vi "test.add.data.to.buffer.vi"() -> (3 "All Passed":bool)   [LabVIEW 2022 SP3]
uses:
  buffer.test.case.ctl
  data.ctl
  <vilib>/rvi/Emulation/niFpgaGetClockAttributes.vi
  <vilib>/rvi/Emulation/niFpgaSctlEmulationGetInTimedLoop.vi
  <vilib>/rvi/Emulation/niFpgaEmulationReportErrorSimple.vi
  <vilib>/rvi/Emulation/niFpgaCriticalErrorInLSC.vi
panel:
  in  "Test Case #12 - Buffer has 16 elements, Data has 3 elements":T1={"data.valid"=TRUE, "data"={"enabled"=[TRUE, TRUE, TRUE, FALSE, FALSE, FALSE, FALSE, FALSE], "byte"=[1, 2, 3, 4, 5, 6, 7, 0]}, "buffer"=[1234605616436508552, 48057234611961600, 0, 0, 0, 0, 0, 0, 0], "buffer.length"=16, "exp.buffer.value.1"=72623842526232576, "index 1"=2, "exp.buffer.value.2"=0, "index 2"=3, "exp.buffer.length"=19} {"exp.buffer.value.2" format="%.0x"; "index 1" format="%.0x"; "exp.buffer.value.1" format="%.0x"; "buffer" format="%.0x"; "data"."byte" format="%.0x"}
  out "Passed 12":bool
  in  "Test Case #11 - Buffer has 16 elements, Data has 8 elements":T1={"data.valid"=TRUE, "data"={"enabled"=[TRUE, TRUE, TRUE, TRUE, TRUE, TRUE, TRUE, TRUE], "byte"=[1, 2, 3, 4, 5, 6, 7, 8]}, "buffer"=[1234605616436508552, 48057234611961600, 0, 0, 0, 0, 0, 0, 0], "buffer.length"=16, "exp.buffer.value.1"=72623859790382856, "index 1"=2, "exp.buffer.value.2"=0, "index 2"=3, "exp.buffer.length"=24} {"exp.buffer.value.2" format="%.0x"; "index 1" format="%.0x"; "exp.buffer.value.1" format="%.0x"; "buffer" format="%.0x"; "data"."byte" format="%.0x"}
  out "Passed 11":bool
  in  "Test Case #10 - Buffer has 32 elements, Data has 8 elements":T1={"data.valid"=TRUE, "data"={"enabled"=[TRUE, TRUE, TRUE, TRUE, TRUE, TRUE, TRUE, TRUE], "byte"=[34, 255, 255, 255, 255, 255, 255, 255]}, "buffer"=[1234605616436508552, 48057234611961600, 1234605616436508552, 11024811887802974208, 0, 0, 0, 0, 0], "buffer.length"=32, "exp.buffer.value.1"=2522015791327477759, "index 1"=4, "exp.buffer.value.2"=0, "index 2"=5, "exp.buffer.length"=40} {"exp.buffer.value.2" format="%.0x"; "index 1" format="%.0x"; "exp.buffer.value.1" format="%.0x"; "buffer" format="%.0x"; "data"."byte" format="%.0x"}
  out "Passed 10":bool
  in  "Test Case #9 - Buffer has 26 elements, Data has 1 element":T1={"data.valid"=TRUE, "data"={"enabled"=[TRUE, FALSE, FALSE, FALSE, FALSE, FALSE, FALSE, FALSE], "byte"=[34, 255, 255, 255, 255, 255, 255, 255]}, "buffer"=[1234605616436508552, 48057234611961600, 1234605616436508552, 11024811887802974208, 0, 0, 0, 0, 0], "buffer.length"=25, "exp.buffer.value.1"=11034382037011136512, "index 1"=3, "exp.buffer.value.2"=0, "index 2"=4, "exp.buffer.length"=26} {"exp.buffer.value.2" format="%.0x"; "index 1" format="%.0x"; "exp.buffer.value.1" format="%.0x"; "buffer" format="%.0x"; "data"."byte" format="%.0x"}
  out "Passed 9":bool
  in  "Test Case #8 - Buffer has 3 elements, Data has 8 elements 2":T1={"data.valid"=TRUE, "data"={"enabled"=[TRUE, TRUE, TRUE, TRUE, TRUE, TRUE, TRUE, TRUE], "byte"=[34, 51, 68, 85, 102, 119, 136, 170]}, "buffer"=[1234605322945953792, 0, 0, 0, 0, 0, 0, 0, 0], "buffer.length"=3, "exp.buffer.value.1"=1234605469834958182, "index 1"=0, "exp.buffer.value.2"=8613321204322795520, "index 2"=1, "exp.buffer.length"=11} {"exp.buffer.value.2" format="%.0x"; "index 1" format="%.0x"; "exp.buffer.value.1" format="%.0x"; "buffer" format="%.0x"; "data"."byte" format="%.0x"}
  out "Passed 8":bool
  in  "Test Case #7 - Buffer has 3 elements, Data has 8 elements":T1={"data.valid"=TRUE, "data"={"enabled"=[TRUE, TRUE, TRUE, TRUE, TRUE, TRUE, TRUE, TRUE], "byte"=[34, 51, 68, 85, 102, 119, 136, 170]}, "buffer"=[1234605322945953792, 0, 0, 0, 0, 0, 0, 0, 0], "buffer.length"=3, "exp.buffer.value.1"=1234605469834958182, "index 1"=0, "exp.buffer.value.2"=8613321204322795520, "index 2"=1, "exp.buffer.length"=11} {"exp.buffer.value.2" format="%.0x"; "index 1" format="%.0x"; "exp.buffer.value.1" format="%.0x"; "buffer" format="%.0x"; "data"."byte" format="%.0x"}
  out "Passed 7":bool
  in  "Test Case #6 - Buffer has 3 elements, Data has 1 element":T1={"data.valid"=TRUE, "data"={"enabled"=[TRUE, FALSE, FALSE, FALSE, FALSE, FALSE, FALSE, FALSE], "byte"=[68, 255, 255, 255, 255, 255, 255, 255]}, "buffer"=[1234605322945953792, 0, 0, 0, 0, 0, 0, 0, 0], "buffer.length"=3, "exp.buffer.value.1"=1234605615003729920, "index 1"=0, "exp.buffer.value.2"=0, "index 2"=1, "exp.buffer.length"=4} {"exp.buffer.value.2" format="%.0x"; "index 1" format="%.0x"; "exp.buffer.value.1" format="%.0x"; "buffer" format="%.0x"; "data"."byte" format="%.0x"}
  out "Passed 6":bool
  in  "Test Case #5 - Buffer has 1 element, Data has 8 elements":T1={"data.valid"=TRUE, "data"={"enabled"=[TRUE, TRUE, TRUE, TRUE, TRUE, TRUE, TRUE, TRUE], "byte"=[34, 51, 68, 85, 102, 119, 136, 170]}, "buffer"=[1224979098644774912, 0, 0, 0, 0, 0, 0, 0, 0], "buffer.length"=1, "exp.buffer.value.1"=1234605616436508552, "index 1"=0, "exp.buffer.value.2"=12249790986447749120, "index 2"=1, "exp.buffer.length"=9} {"exp.buffer.value.2" format="%.0x"; "index 1" format="%.0x"; "exp.buffer.value.1" format="%.0x"; "buffer" format="%.0x"; "data"."byte" format="%.0x"}
  out "Passed 5":bool
  in  "Test #":i16=10
  in  "Override":bool
  out "Passed 4":bool
  in  "Test Case #4 - Buffer has 1 element, Data has 7 elements":T1={"data.valid"=TRUE, "data"={"enabled"=[TRUE, TRUE, TRUE, TRUE, TRUE, TRUE, TRUE, FALSE], "byte"=[34, 51, 68, 85, 102, 119, 136, 255]}, "buffer"=[1224979098644774912, 0, 0, 0, 0, 0, 0, 0, 0], "buffer.length"=1, "exp.buffer.value.1"=1234605616436508552, "index 1"=0, "exp.buffer.value.2"=0, "index 2"=1, "exp.buffer.length"=8} {"exp.buffer.value.2" format="%.0x"; "index 1" format="%.0x"; "exp.buffer.value.1" format="%.0x"; "buffer" format="%.0x"; "data"."byte" format="%.0x"}
  out "Passed 3":bool
  in  "Test Case #3 - Buffer has 1 element, Data has 5 elements":T1={"data.valid"=TRUE, "data"={"enabled"=[TRUE, TRUE, TRUE, TRUE, TRUE, FALSE, FALSE, FALSE], "byte"=[34, 51, 68, 85, 102, 255, 255, 255]}, "buffer"=[1224979098644774912, 0, 0, 0, 0, 0, 0, 0, 0], "buffer.length"=1, "exp.buffer.value.1"=1234605616436477952, "index 1"=0, "exp.buffer.value.2"=0, "index 2"=1, "exp.buffer.length"=6} {"exp.buffer.value.2" format="%.0x"; "index 1" format="%.0x"; "exp.buffer.value.1" format="%.0x"; "buffer" format="%.0x"; "data"."byte" format="%.0x"}
  out "Passed 2":bool
  in  "Test Case #2 - Buffer is Empty, Data has 5 elements":T1={"data.valid"=TRUE, "data"={"enabled"=[TRUE, TRUE, TRUE, TRUE, TRUE, FALSE, FALSE, FALSE], "byte"=[17, 34, 51, 68, 85, 255, 255, 255]}, "buffer"=[0, 0, 0, 0, 0, 0, 0, 0, 0], "buffer.length"=0, "exp.buffer.value.1"=1234605616429793280, "index 1"=0, "exp.buffer.value.2"=0, "index 2"=1, "exp.buffer.length"=5} {"exp.buffer.value.2" format="%.0x"; "index 1" format="%.0x"; "exp.buffer.value.1" format="%.0x"; "buffer" format="%.0x"; "data"."byte" format="%.0x"}
  out "Passed 1":bool
  in  "Test Case #1 - Buffer is Empty, Data has 8 elements":T1={"data.valid"=TRUE, "data"={"enabled"=[TRUE, TRUE, TRUE, TRUE, TRUE, TRUE, TRUE, TRUE], "byte"=[17, 34, 51, 68, 85, 102, 119, 136]}, "buffer"=[0, 0, 0, 0, 0, 0, 0, 0, 0], "buffer.length"=0, "exp.buffer.value.1"=1234605616436508552, "index 1"=0, "exp.buffer.value.2"=0, "index 2"=1, "exp.buffer.length"=8} {"exp.buffer.value.2" format="%.0x"; "index 1" format="%.0x"; "exp.buffer.value.1" format="%.0x"; "buffer" format="%.0x"; "data"."byte" format="%.0x"}
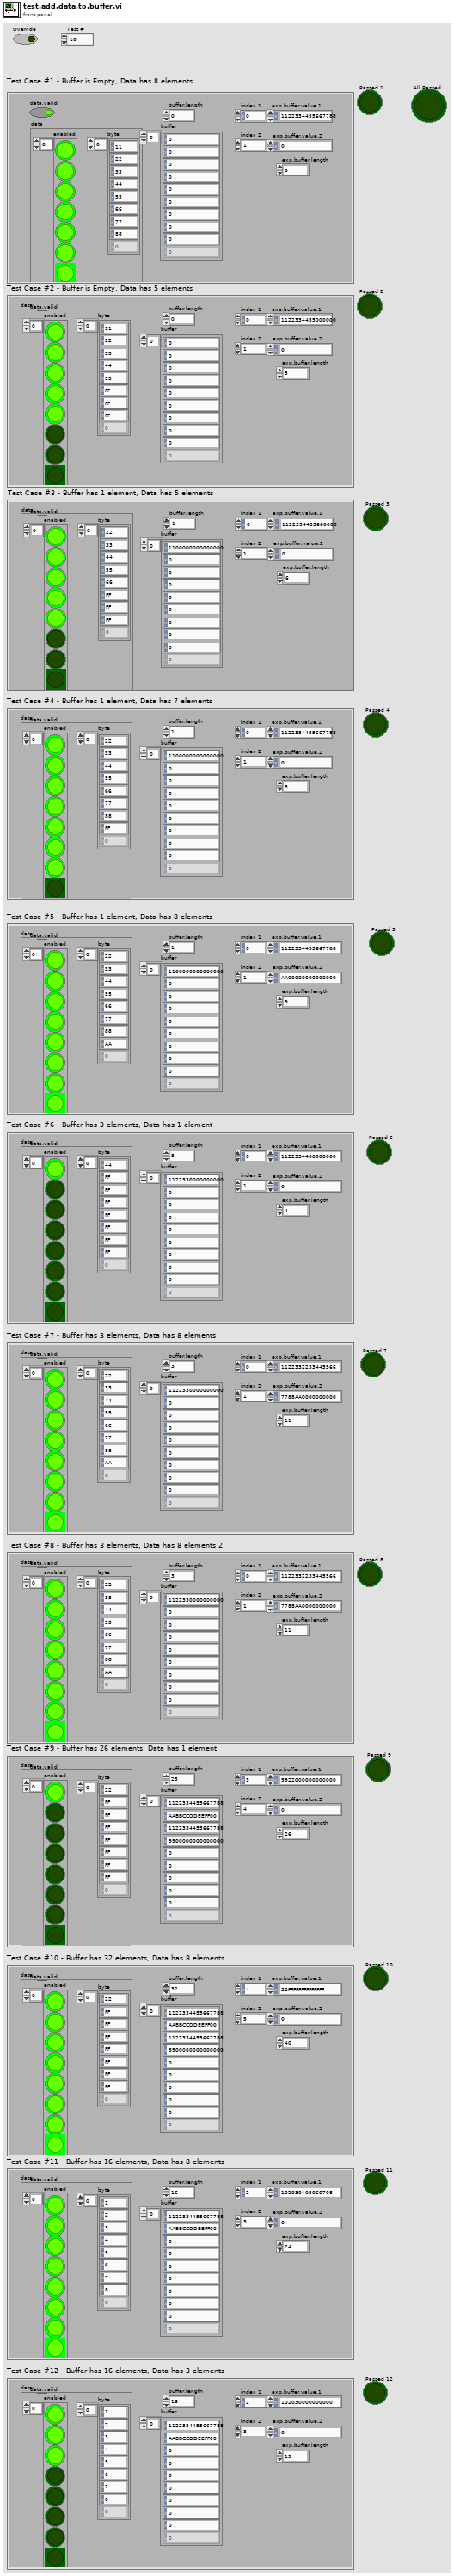
[diagram p1: front panel]
types:
  T1 = typedef "buffer.test.case.ctl" = cluster{"data.valid":bool, "data":T2, "buffer":u64[], "buffer.length":u8, "exp.buffer.value.1":u64, "index 1":i16, "exp.buffer.value.2":u64, "index 2":i16, "exp.buffer.length":u8}
  T2 = typedef "data.ctl" = cluster{"enabled":bool[], "byte":u8[]}
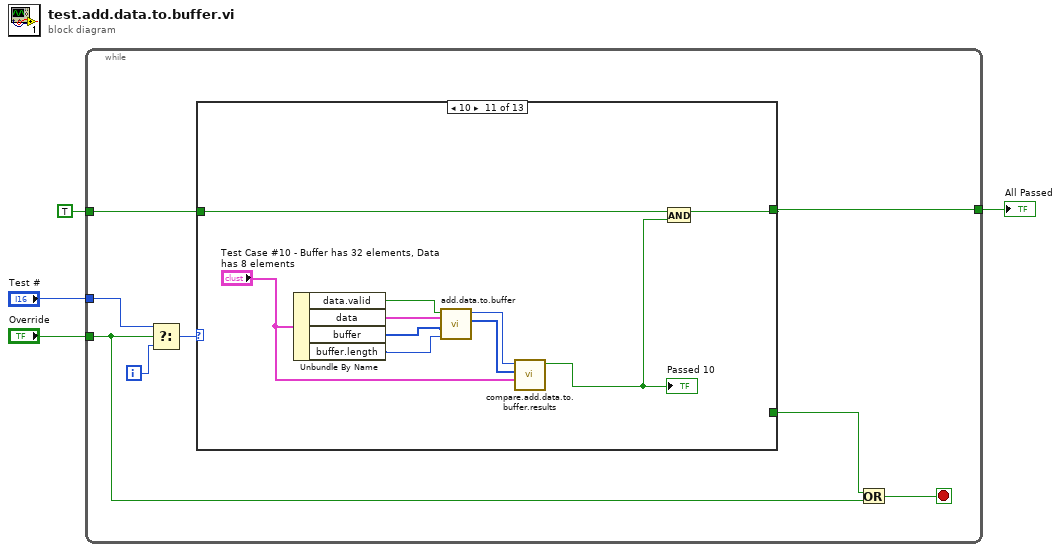
[diagram p0: block diagram]
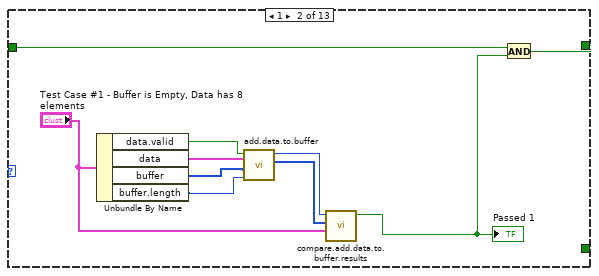
[diagram p3: hidden frame]
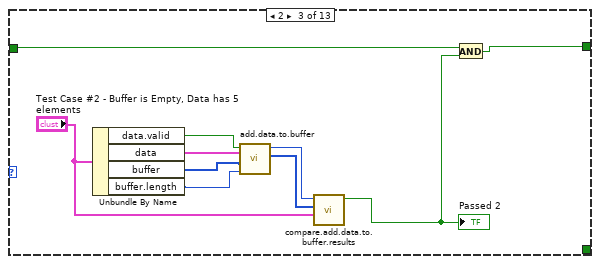
[diagram p4: hidden frame]
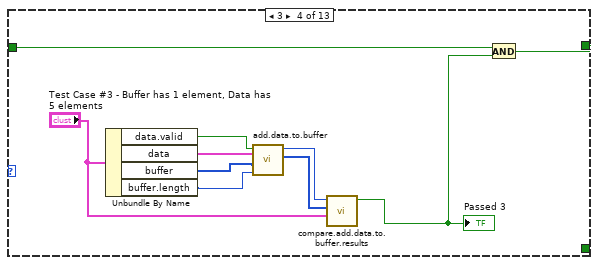
[diagram p5: hidden frame]
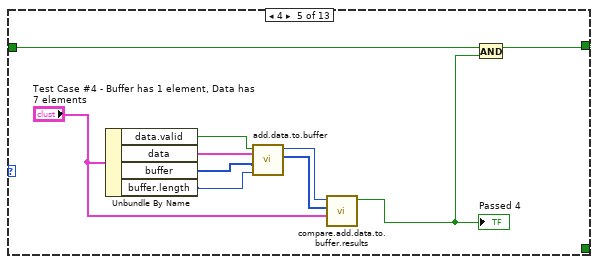
[diagram p6: hidden frame]
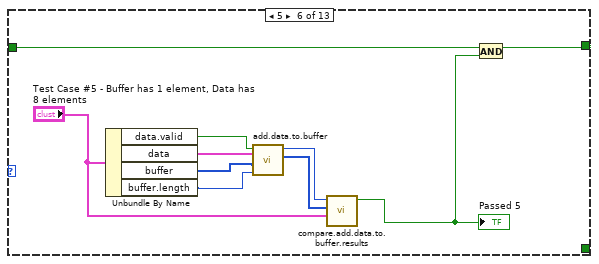
[diagram p7: hidden frame]
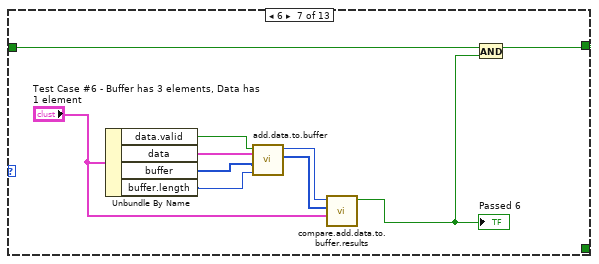
[diagram p8: hidden frame]
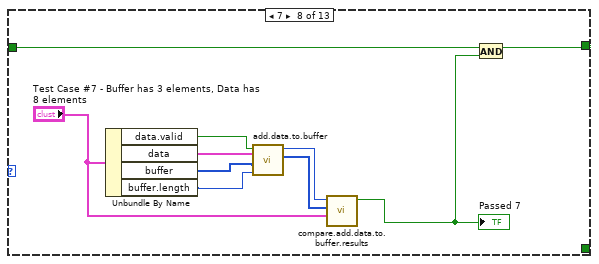
[diagram p9: hidden frame]
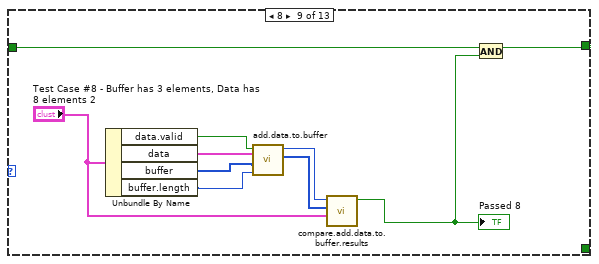
[diagram p10: hidden frame]
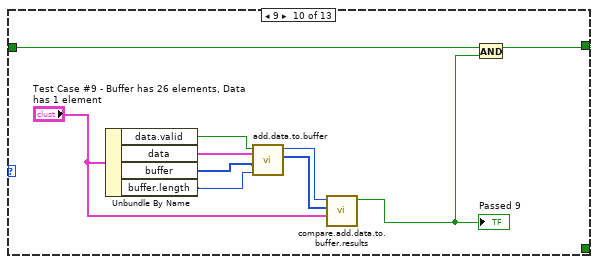
[diagram p11: hidden frame]
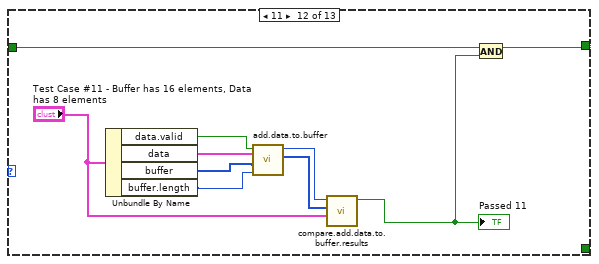
[diagram p12: hidden frame]
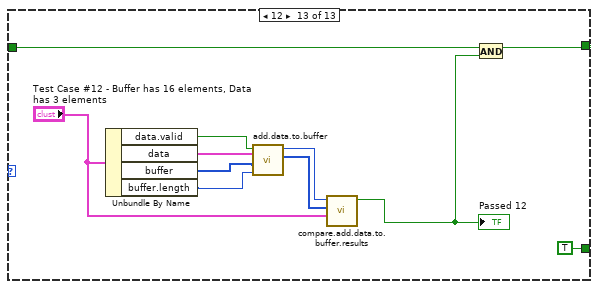
[diagram p13: hidden frame]
diagram:
  n1 = while {
    tunnel: TRUE -> [w11]
    tunnel: [w10] -> w3
    tunnel: "Test #" -> [w9]
    tunnel: "Override" -> [w5]
    i -> [w8]
    stop <- w6 stop-if-true
    n2 = Select(t=w9, s=w5, f=w8) -> (s? t:f=w7:i32)
    n3 = case shown="10" w7 {
      tunnel: [_ _ _ _ _ _ _ _ _ _ _ _ TRUE] -> w12
      tunnel: w11 -> [w13 w14 w26 w35 w47 w57 w67 w77 w87 w97 w107 w117 w128]
      tunnel: [w13 w16 w25 w36 w45 w55 w65 w75 w85 w95 w105 w115 w126] -> w10
      frame 0, Default {
      }
      frame 1 {
        n4 = Unbundle By Name("Test Case #1 - Buffer is Empty, Data has 8 elements") -> ("data.valid"=w20:bool, "data"=w19:T2, "buffer"=w18:u64[], "buffer.length"=w17:u8)
        n5 = call "add.data.to.buffer.vi"("buffer.length"=w17, "buffer"=w18, "data"=w19, "data.valid"=w20) -> ("buffer.out"=w22:u64[], "buffer.length.out"=w23:u8)  [unwired: 6 in]
        n6 = call "compare.add.data.to.buffer.results.vi"("Test Case"="Test Case #1 - Buffer is Empty, Data has 8 elements", "buffer.out"=w22, "buffer.length.out"=w23) -> ("All Passed"=w15:bool)  [unwired: 8 in]
        "Passed 1" <- w15
        n7 = And(x=w14, y=w15) -> (x .and. y?=w16:bool)
      }
      frame 2 {
        n8 = Unbundle By Name("Test Case #2 - Buffer is Empty, Data has 5 elements") -> ("data.valid"=w30:bool, "data"=w29:T2, "buffer"=w28:u64[], "buffer.length"=w27:u8)
        n9 = call "add.data.to.buffer.vi"("buffer.length"=w27, "buffer"=w28, "data"=w29, "data.valid"=w30) -> ("buffer.out"=w32:u64[], "buffer.length.out"=w31:u8)  [unwired: 6 in]
        n10 = call "compare.add.data.to.buffer.results.vi"("Test Case"="Test Case #2 - Buffer is Empty, Data has 5 elements", "buffer.out"=w32, "buffer.length.out"=w31) -> ("All Passed"=w24:bool)  [unwired: 8 in]
        "Passed 2" <- w24
        n11 = And(x=w26, y=w24) -> (x .and. y?=w25:bool)
      }
      frame 3 {
        n12 = Unbundle By Name("Test Case #3 - Buffer has 1 element, Data has 5 elements") -> ("data.valid"=w40:bool, "data"=w39:T2, "buffer"=w38:u64[], "buffer.length"=w37:u8)
        n13 = call "add.data.to.buffer.vi"("buffer.length"=w37, "buffer"=w38, "data"=w39, "data.valid"=w40) -> ("buffer.out"=w42:u64[], "buffer.length.out"=w41:u8)  [unwired: 6 in]
        n14 = call "compare.add.data.to.buffer.results.vi"("Test Case"="Test Case #3 - Buffer has 1 element, Data has 5 elements", "buffer.out"=w42, "buffer.length.out"=w41) -> ("All Passed"=w34:bool)  [unwired: 8 in]
        "Passed 3" <- w34
        n15 = And(x=w35, y=w34) -> (x .and. y?=w36:bool)
      }
      frame 4 {
        n16 = Unbundle By Name("Test Case #4 - Buffer has 1 element, Data has 7 elements") -> ("data.valid"=w51:bool, "data"=w50:T2, "buffer"=w49:u64[], "buffer.length"=w48:u8)
        n17 = call "add.data.to.buffer.vi"("buffer.length"=w48, "buffer"=w49, "data"=w50, "data.valid"=w51) -> ("buffer.out"=w53:u64[], "buffer.length.out"=w52:u8)  [unwired: 6 in]
        n18 = call "compare.add.data.to.buffer.results.vi"("Test Case"="Test Case #4 - Buffer has 1 element, Data has 7 elements", "buffer.out"=w53, "buffer.length.out"=w52) -> ("All Passed"=w44:bool)  [unwired: 8 in]
        "Passed 4" <- w44
        n19 = And(x=w47, y=w44) -> (x .and. y?=w45:bool)
      }
      frame 5 {
        n20 = Unbundle By Name("Test Case #5 - Buffer has 1 element, Data has 8 elements") -> ("data.valid"=w61:bool, "data"=w60:T2, "buffer"=w59:u64[], "buffer.length"=w58:u8)
        n21 = call "add.data.to.buffer.vi"("buffer.length"=w58, "buffer"=w59, "data"=w60, "data.valid"=w61) -> ("buffer.out"=w63:u64[], "buffer.length.out"=w62:u8)  [unwired: 6 in]
        n22 = call "compare.add.data.to.buffer.results.vi"("Test Case"="Test Case #5 - Buffer has 1 element, Data has 8 elements", "buffer.out"=w63, "buffer.length.out"=w62) -> ("All Passed"=w54:bool)  [unwired: 8 in]
        "Passed 5" <- w54
        n23 = And(x=w57, y=w54) -> (x .and. y?=w55:bool)
      }
      frame 6 {
        n24 = Unbundle By Name("Test Case #6 - Buffer has 3 elements, Data has 1 element") -> ("data.valid"=w71:bool, "data"=w70:T2, "buffer"=w69:u64[], "buffer.length"=w68:u8)
        n25 = call "add.data.to.buffer.vi"("buffer.length"=w68, "buffer"=w69, "data"=w70, "data.valid"=w71) -> ("buffer.out"=w73:u64[], "buffer.length.out"=w72:u8)  [unwired: 6 in]
        n26 = call "compare.add.data.to.buffer.results.vi"("Test Case"="Test Case #6 - Buffer has 3 elements, Data has 1 element", "buffer.out"=w73, "buffer.length.out"=w72) -> ("All Passed"=w64:bool)  [unwired: 8 in]
        "Passed 6" <- w64
        n27 = And(x=w67, y=w64) -> (x .and. y?=w65:bool)
      }
      frame 7 {
        n28 = Unbundle By Name("Test Case #7 - Buffer has 3 elements, Data has 8 elements") -> ("data.valid"=w81:bool, "data"=w80:T2, "buffer"=w79:u64[], "buffer.length"=w78:u8)
        n29 = call "add.data.to.buffer.vi"("buffer.length"=w78, "buffer"=w79, "data"=w80, "data.valid"=w81) -> ("buffer.out"=w83:u64[], "buffer.length.out"=w82:u8)  [unwired: 6 in]
        n30 = call "compare.add.data.to.buffer.results.vi"("Test Case"="Test Case #7 - Buffer has 3 elements, Data has 8 elements", "buffer.out"=w83, "buffer.length.out"=w82) -> ("All Passed"=w74:bool)  [unwired: 8 in]
        "Passed 7" <- w74
        n31 = And(x=w77, y=w74) -> (x .and. y?=w75:bool)
      }
      frame 8 {
        n32 = Unbundle By Name("Test Case #8 - Buffer has 3 elements, Data has 8 elements 2") -> ("data.valid"=w91:bool, "data"=w90:T2, "buffer"=w89:u64[], "buffer.length"=w88:u8)
        n33 = call "add.data.to.buffer.vi"("buffer.length"=w88, "buffer"=w89, "data"=w90, "data.valid"=w91) -> ("buffer.out"=w93:u64[], "buffer.length.out"=w92:u8)  [unwired: 6 in]
        n34 = call "compare.add.data.to.buffer.results.vi"("Test Case"="Test Case #8 - Buffer has 3 elements, Data has 8 elements 2", "buffer.out"=w93, "buffer.length.out"=w92) -> ("All Passed"=w84:bool)  [unwired: 8 in]
        "Passed 8" <- w84
        n35 = And(x=w87, y=w84) -> (x .and. y?=w85:bool)
      }
      frame 9 {
        n36 = Unbundle By Name("Test Case #9 - Buffer has 26 elements, Data has 1 element") -> ("data.valid"=w101:bool, "data"=w100:T2, "buffer"=w99:u64[], "buffer.length"=w98:u8)
        n37 = call "add.data.to.buffer.vi"("buffer.length"=w98, "buffer"=w99, "data"=w100, "data.valid"=w101) -> ("buffer.out"=w103:u64[], "buffer.length.out"=w102:u8)  [unwired: 6 in]
        n38 = call "compare.add.data.to.buffer.results.vi"("Test Case"="Test Case #9 - Buffer has 26 elements, Data has 1 element", "buffer.out"=w103, "buffer.length.out"=w102) -> ("All Passed"=w94:bool)  [unwired: 8 in]
        "Passed 9" <- w94
        n39 = And(x=w97, y=w94) -> (x .and. y?=w95:bool)
      }
      frame 10 {
        n40 = Unbundle By Name("Test Case #10 - Buffer has 32 elements, Data has 8 elements") -> ("data.valid"=w111:bool, "data"=w110:T2, "buffer"=w109:u64[], "buffer.length"=w108:u8)
        n41 = call "add.data.to.buffer.vi"("buffer.length"=w108, "buffer"=w109, "data"=w110, "data.valid"=w111) -> ("buffer.out"=w113:u64[], "buffer.length.out"=w112:u8)  [unwired: 6 in]
        n42 = call "compare.add.data.to.buffer.results.vi"("Test Case"="Test Case #10 - Buffer has 32 elements, Data has 8 elements", "buffer.out"=w113, "buffer.length.out"=w112) -> ("All Passed"=w104:bool)  [unwired: 8 in]
        "Passed 10" <- w104
        n43 = And(x=w107, y=w104) -> (x .and. y?=w105:bool)
      }
      frame 11 {
        n44 = Unbundle By Name("Test Case #11 - Buffer has 16 elements, Data has 8 elements") -> ("data.valid"=w121:bool, "data"=w120:T2, "buffer"=w119:u64[], "buffer.length"=w118:u8)
        n45 = call "add.data.to.buffer.vi"("buffer.length"=w118, "buffer"=w119, "data"=w120, "data.valid"=w121) -> ("buffer.out"=w123:u64[], "buffer.length.out"=w122:u8)  [unwired: 6 in]
        n46 = call "compare.add.data.to.buffer.results.vi"("Test Case"="Test Case #11 - Buffer has 16 elements, Data has 8 elements", "buffer.out"=w123, "buffer.length.out"=w122) -> ("All Passed"=w114:bool)  [unwired: 8 in]
        "Passed 11" <- w114
        n47 = And(x=w117, y=w114) -> (x .and. y?=w115:bool)
      }
      frame 12 {
        n48 = Unbundle By Name("Test Case #12 - Buffer has 16 elements, Data has 3 elements") -> ("data.valid"=w132:bool, "data"=w131:T2, "buffer"=w130:u64[], "buffer.length"=w129:u8)
        n49 = call "add.data.to.buffer.vi"("buffer.length"=w129, "buffer"=w130, "data"=w131, "data.valid"=w132) -> ("buffer.out"=w134:u64[], "buffer.length.out"=w133:u8)  [unwired: 6 in]
        n50 = call "compare.add.data.to.buffer.results.vi"("Test Case"="Test Case #12 - Buffer has 16 elements, Data has 3 elements", "buffer.out"=w134, "buffer.length.out"=w133) -> ("All Passed"=w125:bool)  [unwired: 8 in]
        "Passed 12" <- w125
        n51 = And(x=w128, y=w125) -> (x .and. y?=w126:bool)
      }
    }
    n52 = Or(x=w12, y=w5) -> (x .or. y?=w6:bool)
  }
  "All Passed" <- w3
